vi "Setup UI.vi"(8 "error in (no error)":errorcluster, 10 "Set UI to input? (F)":bool, 11 "Lockin SR830 in":refnum<class "Lockin SR830.lvclass">) -> (0 "error out":errorcluster, 3 "Lockin SR830 out":refnum<class "Lockin SR830.lvclass">)   [LabVIEW 2012, in "Lockin SR830.lvclass"]
doc: "Setup UI constructs an object -- populates its member data -- from a front panel the user can see. The VI should be as simple as possible so that a UI loop can poll it continuously for updates. \n\nThe VI is designed to be used as a subPanel within another VI. Wire true to \"Set UI to input\" only on the first call, just after inserting this VI into a subPanel, to populate its controls with the class's current values.\n\nSetup UI is distinct from the class constructor. Class constructors are not polymorphic, yet configure dialogs need to configure objects without knowing their type -- and polymorphism is the necessary solution. Thus, Setup UI is a polymorphic class constructor. This continously polled \"Setup UI\" concept is a kludge: a better idea would be an XControl, but those require a steeper learning curve."
uses:
  Lockin SR830.lvclass
  Sensitivity.ctl
  Utility Classes/Readable/Readable.lvclass
panel:
  in  "Set Parameters":bool
  in  "Sensitivity":T1 items=["2 nV", "5 nV", "10 nV", "20 nV", "50 nV", "100 nV", "200 nV", "500 nV", "1 uV", "2 uV", "5 uV", "10 uV", "20 uV", "50 uV", "100 uV", "200 uV", "500 uV", "1 mV", "2 mV", "5 mV", "10 mV", "20 mV", "50 mV", "100 mV", "200 mV", "500 mV", "1 V"]
  in  "Tau":u16(ring) items=["10 us", "30 us", "100 us", "300 us", "1 ms", "3 ms", "10 ms", "30 ms", "100 ms", "300 ms", "1 s", "3 s", "10 s", "30 s", "100 s", "300 s", "1 ks", "3 ks", "10 ks", "30 ks"]
  in  "Using Lockin":bool=TRUE
  # "Lockin Setup"
  # "SR810"
  # "SR830"
  # "GPIB #8"
  # "GPIB #9"
  # "Takes data from X, Y, and R channels."
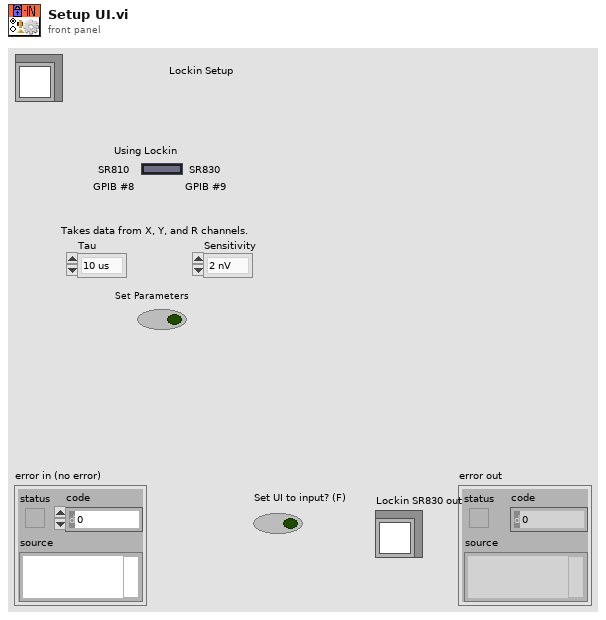
[diagram p1: front panel]
types:
  T1 = typedef "Lockin SR830.lvclass/Sensitivity.ctl" = u16
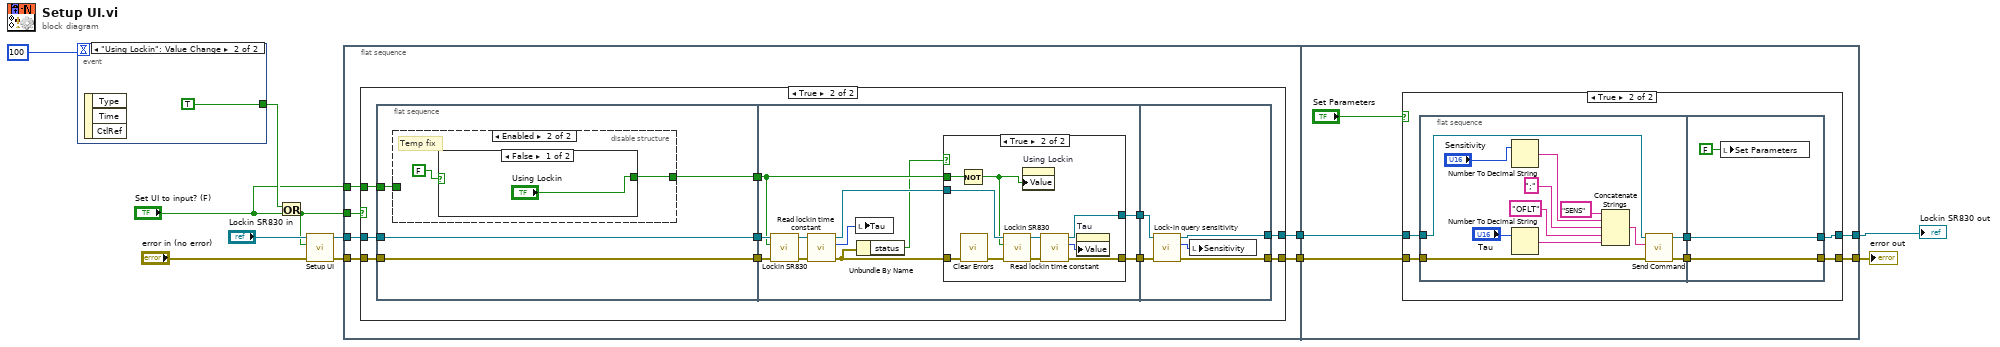
[diagram p0: block diagram]
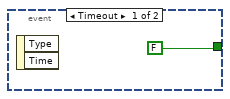
[diagram p2: hidden frame]
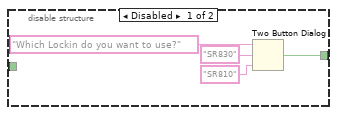
[diagram p4: hidden frame]
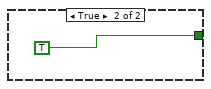
[diagram p5: hidden frame]
diagram:
  n1 = event shown="[1] \"Using Lockin\": Value Change" {
    selector: _ -> [_ _]
    dyn-events: _ -> [_ _]
    timeout: 100 -> [_ _]
    tunnel: [FALSE TRUE] -> w2
    event Timeout {
      n2 = event-data() -> ()  [unwired: 1 in, 2 out]
    }
    event "Using Lockin": Value Change {
      n3 = event-data() -> ()  [unwired: 1 in, 3 out]
    }
  }
  n4 = Or(x=w2, y="Set UI to input? (F)") -> (x .or. y?=w4:bool)
  n5 = call-parent "Setup UI.vi"("error in (no error)"="error in (no error)", "Set UI to input? (F)"=w4, "Instrument in"="Lockin SR830 in") -> ("error out"=w6:errorcluster, "Instrument out"=w5:refnum<class "Lockin SR830.lvclass">)  [unwired: 7 out]
  n6 = flat-sequence {
    tunnel: w6 -> [w20]
    tunnel: w5 -> [w17]
    tunnel: w4 -> [w16]
    tunnel: [w19] -> w10
    tunnel: [w18] -> w9
    tunnel: "Set UI to input? (F)" -> [w15]
    tunnel: [w74] -> w11
    tunnel: [w76] -> w12
    tunnel: w10 -> [w77]
    tunnel: w9 -> [w75]
    frame #0 {
      n7 = case shown="True" w16 {
        tunnel: w20 -> [w21 w32]
        tunnel: [w22 w30] -> w19
        tunnel: [w21 w29] -> w18
        tunnel: w17 -> [w22 w31]
        tunnel: w15 -> [_ w23]
        frame False {
        }
        frame True {
          n8 = flat-sequence {
            tunnel: w31 -> [w36]
            tunnel: w32 -> [w35]
            tunnel: [w36] -> w28
            tunnel: [w35] -> w27
            tunnel: [w34] -> w26
            tunnel: w23 -> [w33]
            tunnel: w28 -> [w54]
            tunnel: w27 -> [w53]
            tunnel: w26 -> [w46]
            tunnel: [w51] -> w25
            tunnel: [w48] -> w24
            tunnel: [w71] -> w30
            tunnel: [w70] -> w29
            tunnel: w25 -> [w69]
            tunnel: w24 -> [w68]
            frame #0 {
              n9 = disable-structure shown="Enabled" {
                disable-tunnel: [w37 w42] -> w34
                disable-tunnel: w33 -> [_ _]
                frame Disabled {
                  n10 = Two Button Dialog(message="Which Lockin do you want to use?", 1:"SR810" ("F button name (\"Cancel\")"), 2:"SR830" ("T button name (\"OK\")")) -> (T button?=w37:bool)
                }
                frame Enabled {
                  # "Temp fix"
                  n11 = case shown="False" FALSE {
                    tunnel: ["Using Lockin" TRUE] -> w42
                    frame False {
                    }
                    frame True {
                    }
                  }
                }
              }
            }
            frame #1 {
              n12 = call "Lockin SR830.vi"("error in (no error)"=w53, "Is SR830? (T)"=w46, "Lockin SR830 in"=w54) -> ("error out"=w52:errorcluster, "Lockin SR830 out"=w50:refnum<class "Lockin SR830.lvclass">)  [unwired: 7 out]
              n13 = call "Read lockin time constant.vi"("error in (no error)"=w52, "Lockin SR830.lvclass In"=w50) -> ("error out"=w47:errorcluster, "Tau"=w55:u16, "Lockin SR830.lvclass out"=w49:refnum<class "Lockin SR830.lvclass">)  [unwired: 7 in]
              n14 = local write "Tau"(w55) -> ()
              n15 = Unbundle By Name(w47) -> ("status"=w45:bool)
              n16 = case shown="True" w45 {
                tunnel: [w56 w62] -> w51
                tunnel: w49 -> [w57 w66]
                tunnel: [w57 w60] -> w48
                tunnel: w46 -> [_ w67]
                tunnel: w47 -> [w56 w59]
                frame False {
                }
                frame True {
                  n17 = Not(x=w67) -> (.not. x?=w58:bool)
                  n18 = call <vilib>:"Clear Errors.vi"("error in (no error)"=w59) -> ("error out"=w63:errorcluster)  [unwired: 6 in]
                  n19 = call "Lockin SR830.vi"("error in (no error)"=w63, "Is SR830? (T)"=w58, "Lockin SR830 in"=w66) -> ("error out"=w65:errorcluster, "Lockin SR830 out"=w64:refnum<class "Lockin SR830.lvclass">)  [unwired: 7 out]
                  n20 = property on="Using Lockin" class="Bool (strict)"("Value"=w58) -> ()  [unwired: 2 in, 2 out]
                  n21 = call "Read lockin time constant.vi"("error in (no error)"=w65, "Lockin SR830.lvclass In"=w64) -> ("error out"=w62:errorcluster, "Tau"=w61:u16, "Lockin SR830.lvclass out"=w60:refnum<class "Lockin SR830.lvclass">)  [unwired: 7 in]
                  n22 = property on="Tau" class="Ring (strict)"("Value"=w61) -> ()  [unwired: 2 in, 2 out]
                }
              }
            }
            frame #2 {
              n23 = call "Lock-in query sensitivity.vi"("error in (no error)"=w69, "Lockin SR830.lvclass In"=w68) -> ("error out"=w70:errorcluster, "Sensitivity"=w72:T1, "Lockin SR830.lvclass out"=w71:refnum<class "Lockin SR830.lvclass">)  [unwired: 7 in]
              n24 = local write "Sensitivity"(w72) -> ()
            }
          }
        }
      }
    }
    frame #1 {
      n25 = case shown="True" "Set Parameters" {
        tunnel: w77 -> [w79 w85]
        tunnel: [w79 w84] -> w76
        tunnel: w75 -> [w78 w83]
        tunnel: [w78 w82] -> w74
        frame False {
        }
        frame True {
          n26 = flat-sequence {
            tunnel: w85 -> [w97]
            tunnel: w83 -> [w95]
            tunnel: [w96] -> w81
            tunnel: [w94] -> w80
            tunnel: [w99] -> w82
            tunnel: [w100] -> w84
            tunnel: w81 -> [w100]
            tunnel: w80 -> [w99]
            frame #0 {
              n27 = Number To Decimal String(number="Sensitivity") -> (decimal integer string=w91:string)  [unwired: 1 in]
              n28 = Number To Decimal String(number="Tau") -> (decimal integer string=w87:string)  [unwired: 1 in]
              n29 = Concatenate Strings("SENS" ("Command String"), w91, ";" ("string"), "OFLT" ("Command String"), w87) -> (w86:string)
              n30 = call "Send Command.vi"("error in (no error)"=w95, "Command String"=w86, "Lockin SR830.lvclass In"=w97) -> ("error out"=w94:errorcluster, "Lockin SR830.lvclass out"=w96:refnum<class "Lockin SR830.lvclass">)  [unwired: 7 in]
            }
            frame #1 {
              n31 = local write "Set Parameters"(FALSE ("Set Parameters")) -> ()
            }
          }
        }
      }
    }
  }
  "error out" <- w11
  "Lockin SR830 out" <- w12
